vi "Teleop.vi"(10 "Match Info":T1={"Autonomous Elapsed Seconds"=0.0, "TeleOp Elapsed Seconds"=0.0, "Disabled Elapsed Seconds"=0.0, "Visited Autonomous"=FALSE, "Visited TeleOp"=FALSE, "Visited Disabled"=FALSE, "Autonomous Settings"={"Autonomous Style"=enum."Independent", "VI Refnum"=refnum}}, 11 "Call Context":T2) -> ()   [LabVIEW 2013]
doc: "This VI is called for each TeleOp packet received from the DS where the robot is not disabled. It is often used to read from the joysticks and update I/O or to update setpoints for timed control loops. It should complete and return within 20 milliseconds or it may miss DS packets."
uses:
  <vilib>/Rock Robotics/WPI/DriverStation/WPI_DriverStationDerivedRobotMode.ctl
  <vilib>/Rock Robotics/WPI/DriverStation/WPI_DriverStationMatch Info.ctl
  <vilib>/Rock Robotics/WPI/Solenoid/WPI_SolenoidValue.ctl
  Robot Global Data.vi
  <vilib>/Rock Robotics/WPI/Solenoid/Deprecated/WPI_SolenoidGetBool.vi
  <vilib>/Rock Robotics/WPI/Solenoid/WPI_SolenoidSetEnum.vi
  <vilib>/Rock Robotics/WPI/Joystick/WPI_JoystickGetSetRefNum.vi
  <vilib>/Rock Robotics/WPI/RobotDrive/WPI_RobotDriveGetSetRefNum.vi
panel:
  out "Numeric 1":dbl(slide) scale=0.0..100.0
  out "Boolean 2":bool
  out "Boolean 1":bool
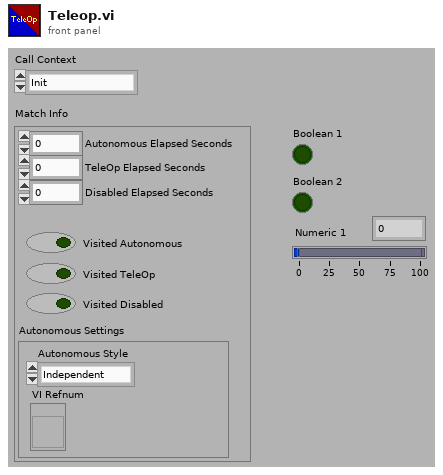
[diagram p1: front panel]
types:
  T1 = typedef "WPI_DriverStationMatch Info.ctl" = cluster{"Autonomous Elapsed Seconds":dbl, "TeleOp Elapsed Seconds":dbl, "Disabled Elapsed Seconds":dbl, "Visited Autonomous":bool, "Visited TeleOp":bool, "Visited Disabled":bool, "Autonomous Settings":cluster{"Autonomous Style":enum16{"Iterative", "Independent"}, "VI Refnum":refnum<vi>}}
  T2 = typedef "WPI_DriverStationDerivedRobotMode.ctl" = enum16{"Init", "Execute", "Stop"}
  T3 = typedef "WPI_JoystickDevRef.ctl" = cluster{"Device":T4}
  T4 = typedef "WPI_JoystickDeviceEnum.ctl" = enum16{"USB 1", "USB 2", "USB 3", "USB 4", "Kinect 1", "Kinect 2"}
  T5 = typedef "WPI_JoystickButtonState.ctl" = cluster{"Button 1":bool, "Button 2":bool, "Button 3":bool, "Button 4":bool, "Button 5":bool, "Button 6":bool, "Button 7":bool, "Button 8":bool, "Button 9":bool, "Button 10":bool, "Button 11":bool, "Button 12":bool}
  T6 = typedef "WPI_SolenoidDevRef.ctl" = cluster{"DevStatus":errorcluster, "Solenoid Module":T7, "Forward Solenoid Channel":T8, "Reverse Solenoid Channel":T8}
  T7 = typedef "FPGA_TypedefSolenoidModule.ctl" = enum16{"Solenoid Module 1", "Solenoid Module 2"}
  T8 = typedef "WPI_SolenoidChannel.ctl" = enum8{"Solenoid 1", "Solenoid 2", "Solenoid 3", "Solenoid 4", "Solenoid 5", "Solenoid 6", "Solenoid 7", "Solenoid 8", "Invalid"}
  T9 = typedef "WPI_SolenoidValue.ctl" = enum16{"Off", "On", "Forward", "Reverse"}
  T10 = typedef "WPI_MotorControlDeviceRef.ctl" = cluster{"DeviceStatus":errorcluster, "Type":enum16{"PWM", "CAN"}, "PWM":cluster{"Digital Module":T11, "PWM Channel":T12, "DeadBand":T13}, "CAN":cluster{"Device Number":u8, "Control Mode":T14, "Semaphore":T15, "Max Vout":dbl}, "Invert":bool, "TransformRef":T16, "InvTransformRef":T16}
  T11 = typedef "FPGA_TypedefDigitalModule.ctl" = enum16{"Digital Module 1", "Digital Module 2"}
  T12 = typedef "FPGA_DIOPWMChannel.ctl" = enum8{"PWM 1", "PWM 2", "PWM 3", "PWM 4", "PWM 5", "PWM 6", "PWM 7", "PWM 8", "PWM 9", "PWM 10", "Invalid"}
  T13 = typedef "WPI_PWMDeadband.ctl" = cluster{"Name":string, "maxPositivePwm":i32, "minPositivePwm":i32, "centerPwm":i32, "maxNegativePwm":i32, "minNegativePwm":i32, "angularRange":u16}
  T14 = typedef "WPI_CANJaguar_ControlMode.ctl" = enum8{"Percent VBus", "Current", "Speed", "Position", "Voltage"}
  T15 = typedef "Semaphore RefNum" = refnum<k1>
  T16 = typedef "WPI_PWMTransform_ConPane.ctl" = refnum<vi>
  T17 = typedef "WPI_RobotDriveDevRef.ctl" = cluster{"DevStatus":errorcluster, "Motors[]":T10[], "Square Inputs":bool, "Max Output":dbl, "Isochronous":bool}
  T18 = cluster{"axis 1 (x)":dbl, "axis 2 (y)":dbl, "axis 3 (throttle)":dbl, "axis 4":dbl, "axis 5":dbl, "axis 6":dbl}
  T19 = typedef "WPI_RelayDevRef.ctl" = cluster{"DevStatus":errorcluster, "Relay Channel":T20, "Digital Module":T11, "Relay Direction":T21}
  T20 = typedef "FPGA_DIORelayChannel.ctl" = enum8{"Relay 1", "Relay 2", "Relay 3", "Relay 4", "Relay 5", "Relay 6", "Relay 7", "Relay 8", "Invalid"}
  T21 = typedef "WPI_RelayDirection.ctl" = enum16{"Both directions", "Forward only", "Reverse only"}
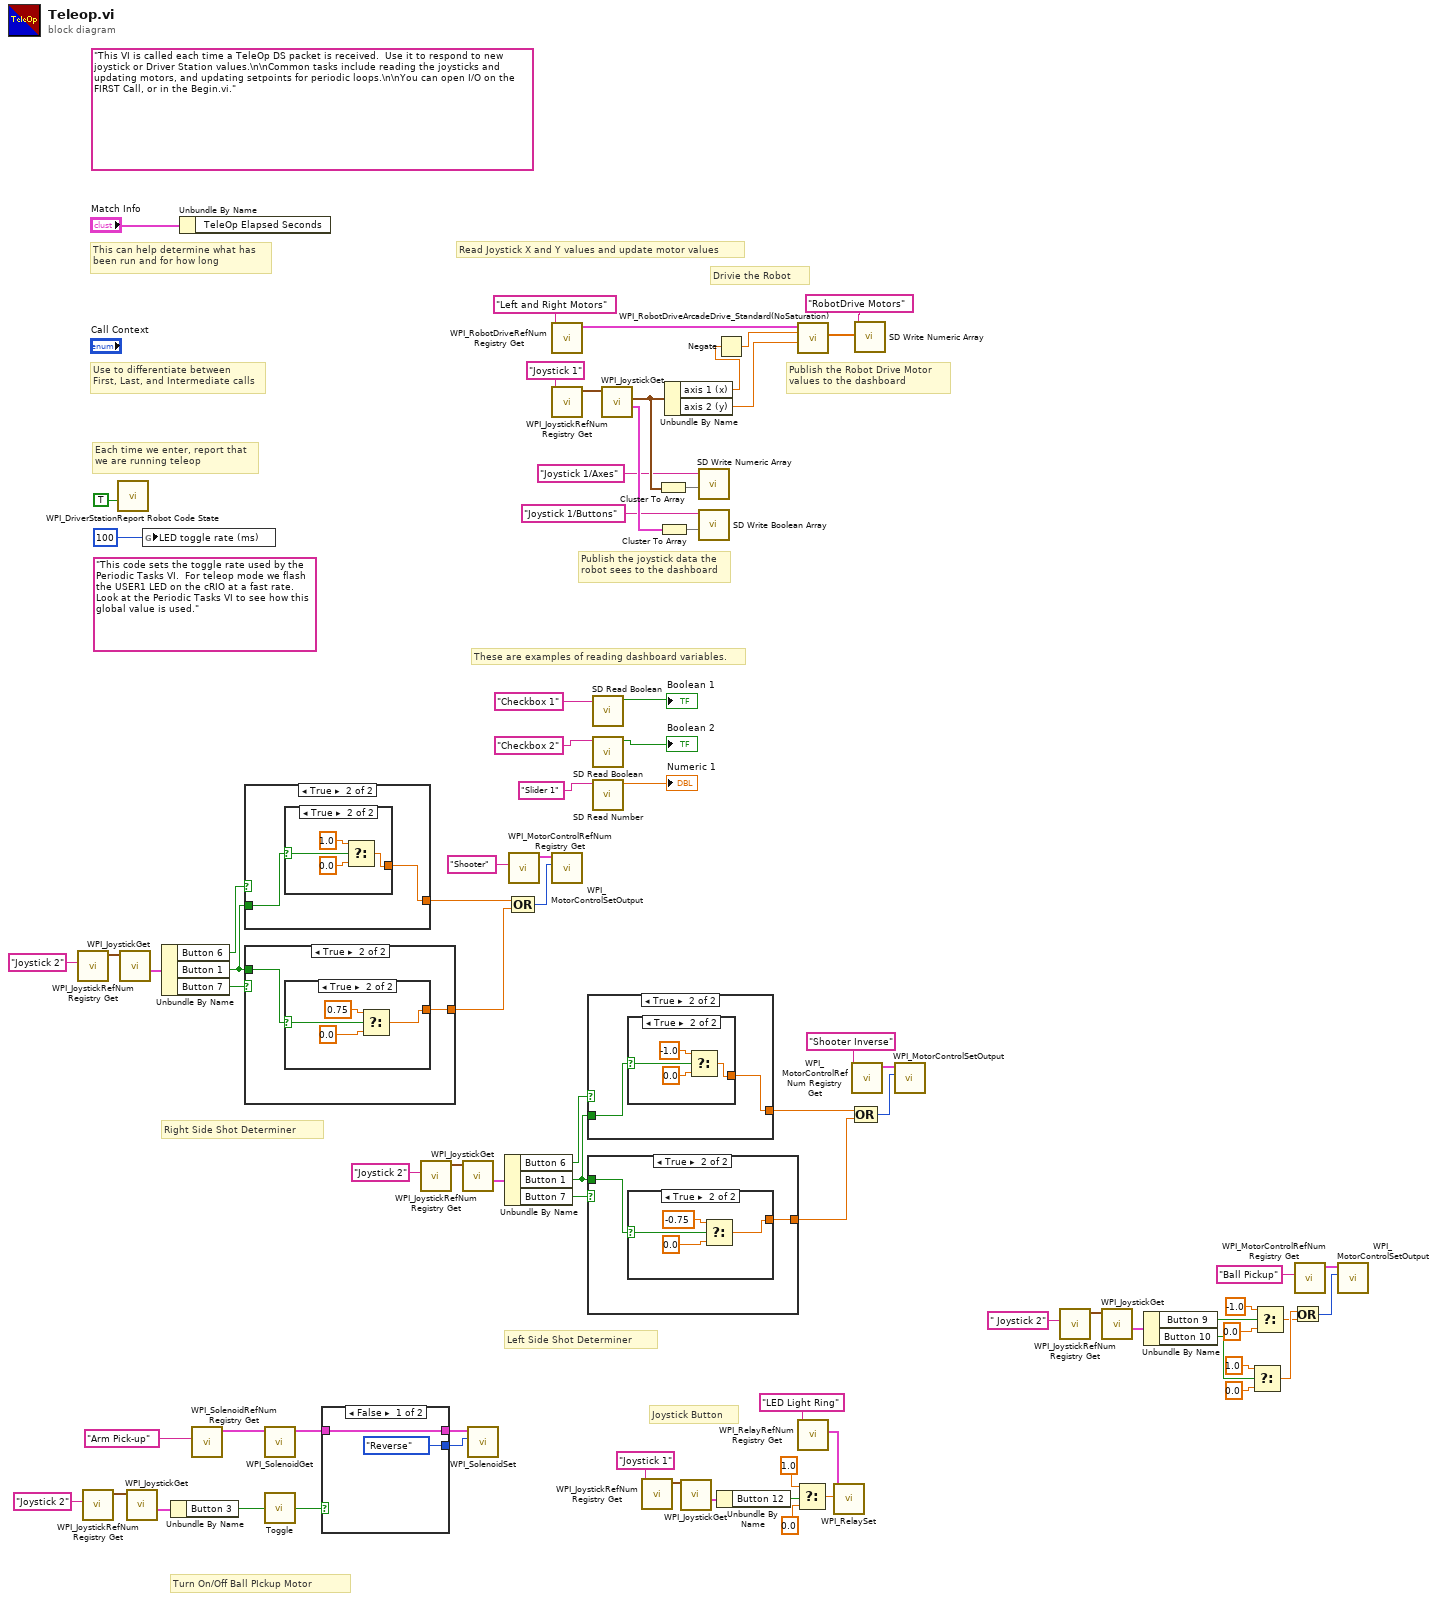
[diagram p0: block diagram]
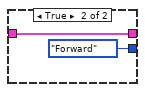
[diagram p2: hidden frame]
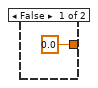
[diagram p3: hidden frame]
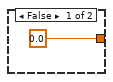
[diagram p4: hidden frame]
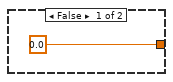
[diagram p5: hidden frame]
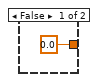
[diagram p6: hidden frame]
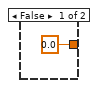
[diagram p7: hidden frame]
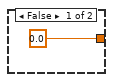
[diagram p8: hidden frame]
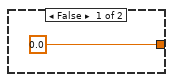
[diagram p9: hidden frame]
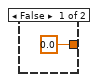
[diagram p10: hidden frame]
diagram:
  (unwired) "This code sets the toggle rate used by the Periodic Tasks VI.  For teleop mode we flash the USER1 LED on the cRIO at a fast rate.  Look at the Periodic Tasks VI to see how this global value is used."
  (unwired) "This VI is called each time a TeleOp DS packet is received.  Use it to respond to new joystick or Driver Station values.\n\nCommon tasks include reading the joysticks and updating motors, and updating setpoints for periodic loops.\n\nYou can open I/O on the FIRST Call, or in the Begin.vi."
  # "Left Side Shot Determiner"
  # "Turn On/Off Ball PIckup Motor"
  # "Right Side Shot Determiner"
  # "Joystick Button"
  # "Drivie the Robot"
  # "These are examples of reading dashboard variables."
  # "Publish the Robot Drive Motor\nvalues to the dashboard"
  # "Publish the joystick data the\nrobot sees to the dashboard"
  # "Each time we enter, report that\nwe are running teleop"
  # "Use to differentiate between\nFirst, Last, and Intermediate calls"
  # "This can help determine what has\nbeen run and for how long"
  # "Read Joystick X and Y values and update motor values"
  n1 = call <vilib>:"WPI_JoystickRefNum Registry Get.vi"("refnum name"="Joystick 2") -> ("JoystickDevRef"=w47:T3)  [unwired: 9 in, 1 out]
  n2 = call <vilib>:"WPI_JoystickRefNum Registry Get.vi"("refnum name"="Joystick 2") -> ("JoystickDevRef"=w41:T3)  [unwired: 9 in, 1 out]
  n3 = call <vilib>:"WPI_DriverStationReport Robot Code State.vi"("TeleOp"=TRUE ("Autonomous")) -> ()  [unwired: 10 in, 1 out]
  n4 = call <vilib>:"WPI_JoystickGet.vi"("JoystickDevRef"=w47) -> ("Buttons"=w46:T5)  [unwired: 4 in, 2 out]
  n5 = call <vilib>:"WPI_JoystickGet.vi"("JoystickDevRef"=w41) -> ("Buttons"=w40:T5)  [unwired: 4 in, 2 out]
  n6 = global write "Robot Global Data.vi" "LED toggle rate (ms)"(u32 100 ("LED ms toggle rate")) -> ()
  n7 = Unbundle By Name(w46) -> ("Button 6"=w36:bool, "Button 1"=w34:bool, "Button 7"=w35:bool)
  n8 = Unbundle By Name(w40) -> ("Button 3"=w37:bool)
  n9 = Unbundle By Name("Match Info") -> ()  [unwired: 1 out]
  n10 = call <vilib>:"WPI_SolenoidRefNum Registry Get.vi"("refnum name"="Arm Pick-up") -> ("SolenoidDevRef"=w5:T6)  [unwired: 9 in, 1 out]
  n11 = case shown="True" w36 {
    tunnel: w34 -> [_ w82]
    tunnel: [0.0 ("f") w81] -> w33
    frame False {
    }
    frame True {
      n12 = case shown="True" w82 {
        selector: w82 -> [_ w85]
        tunnel: [0.0 ("f") w84] -> w81
        frame False {
        }
        frame True {
          n13 = Select(t=1.0, s=w85, f=0.0) -> (s? t:f=w84:dbl)
        }
      }
    }
  }
  n14 = case shown="True" w35 {
    tunnel: w34 -> [_ w90]
    tunnel: [0.0 ("f") w89] -> w32
    frame False {
    }
    frame True {
      n15 = case shown="True" w90 {
        selector: w90 -> [_ w93]
        tunnel: [0.0 ("f") w92] -> w89
        frame False {
        }
        frame True {
          n16 = Select(t=0.75, s=w93, f=0.0) -> (s? t:f=w92:dbl)
        }
      }
    }
  }
  n17 = call-poly <vilib>:"WPI_SolenoidGet.vi"("SolenoidDevRef"=w5) -> ("SolenoidDevRef"=w3:T6)  [unwired: 8 in, 2 out]
  n18 = call "Toggle.vi"("Input"=w37) -> ("Toggled Output"=w4:bool)
  n19 = case shown="False" w4 {
    tunnel: w3 -> [w97 w99]
    tunnel: [w97 w99] -> w2
    tunnel: [WPI_SolenoidValue."Reverse" ("Value") WPI_SolenoidValue."Forward" ("Value")] -> w1
    frame False {
    }
    frame True {
    }
  }
  n20 = call <vilib>:"WPI_JoystickRefNum Registry Get.vi"("refnum name"="Joystick 2") -> ("JoystickDevRef"=w19:T3)  [unwired: 9 in, 1 out]
  n21 = call <vilib>:"WPI_JoystickGet.vi"("JoystickDevRef"=w19) -> ("Buttons"=w20:T5)  [unwired: 4 in, 2 out]
  n22 = call-poly <vilib>:"WPI_SolenoidSet.vi"("Value"=w1, "SolenoidDevRef"=w2) -> ()  [unwired: 8 in, 2 out]
  n23 = Unbundle By Name(w20) -> ("Button 6"=w21:bool, "Button 1"=w23:bool, "Button 7"=w22:bool)
  n24 = call <vilib>:"WPI_MotorControlRefNum Registry Get.vi"("refnum name"="Shooter") -> ("MotorControlDevRef"=w29:T10)  [unwired: 9 in, 1 out]
  n25 = Compound Arithmetic op=OR(w33, w32) -> (w31:i32)
  n26 = call <vilib>:"WPI_RobotDriveRefNum Registry Get.vi"("refnum name"="Left and Right Motors") -> ("RobotDriveDevRef"=w77:T17)  [unwired: 1 in, 9 out]
  n27 = call <vilib>:"WPI_JoystickRefNum Registry Get.vi"("refnum name"="Joystick 1") -> ("JoystickDevRef"=w74:T3)  [unwired: 1 in, 9 out]
  n28 = call <vilib>:"WPI_MotorControlSetOutput.vi"("Output"=w31, "MotorControlDevRef"=w29) -> ()  [unwired: 7 in, 3 out]
  n29 = case shown="True" w21 {
    tunnel: w23 -> [_ w102]
    tunnel: [0.0 ("f") w101] -> w24
    frame False {
    }
    frame True {
      n30 = case shown="True" w102 {
        selector: w102 -> [_ w105]
        tunnel: [0.0 ("f") w104] -> w101
        frame False {
        }
        frame True {
          n31 = Select(t=-1.0, s=w105, f=0.0) -> (s? t:f=w104:dbl)
        }
      }
    }
  }
  n32 = case shown="True" w22 {
    tunnel: w23 -> [_ w110]
    tunnel: [0.0 ("f") w109] -> w25
    frame False {
    }
    frame True {
      n33 = case shown="True" w110 {
        selector: w110 -> [_ w113]
        tunnel: [0.0 ("f") w112] -> w109
        frame False {
        }
        frame True {
          n34 = Select(t=-0.75, s=w113, f=0.0) -> (s? t:f=w112:dbl)
        }
      }
    }
  }
  n35 = call <vilib>:"SD Read Boolean.vi"("Name"="Checkbox 1" ("refnum name")) -> ("Boolean"=→"Boolean 1":bool)  [unwired: 8 in, 2 out]
  n36 = call <vilib>:"SD Read Boolean.vi"("Name"="Checkbox 2" ("refnum name")) -> ("Boolean"=→"Boolean 2":bool)  [unwired: 8 in, 2 out]
  n37 = call <vilib>:"SD Read Number.vi"("Name"="Slider 1" ("refnum name")) -> ("Numeric"=→"Numeric 1":dbl)  [unwired: 8 in, 2 out]
  n38 = call <vilib>:"WPI_JoystickGet.vi"("JoystickDevRef"=w74) -> ("Buttons"=w71:T5, "Axes"=w68:T18)  [unwired: 1 in, 4 out]
  n39 = call <vilib>:"WPI_JoystickRefNum Registry Get.vi"("refnum name"="Joystick 1") -> ("JoystickDevRef"=w53:T3)  [unwired: 9 in, 1 out]
  n40 = Cluster To Array(cluster=w68) -> (array=w67:dbl[])
  n41 = Cluster To Array(cluster=w71) -> (array=w70:bool[])
  n42 = Unbundle By Name(w68) -> ("axis 1 (x)"=w39:dbl, "axis 2 (y)"=w76:dbl)
  n43 = call <vilib>:"WPI_JoystickGet.vi"("JoystickDevRef"=w53) -> ("Buttons"=w52:T5)  [unwired: 4 in, 2 out]
  n44 = call <vilib>:"SD Write Numeric Array.vi"("Numeric Array"=w67, "Name"="Joystick 1/Axes") -> ()  [unwired: 8 in, 2 out]
  n45 = call <vilib>:"SD Write Boolean Array.vi"("Boolean Array"=w70, "Name"="Joystick 1/Buttons") -> ()  [unwired: 8 in, 2 out]
  n46 = Negate(x=w39) -> (-x=w38:dbl)
  n47 = Unbundle By Name(w52) -> ("Button 12"=w51:bool)
  n48 = Select(t=1.0, s=w51, f=0.0) -> (s? t:f=w50:dbl)
  n49 = call <vilib>:"WPI_RobotDriveArcadeDrive_Standard(NoSaturation).vi"("Y axis value"=w76, "X axis value"=w38, "RobotDriveDevRef"=w77) -> ("Motor Values"=w64:dbl[])  [unwired: 1 in, 7 out]
  n50 = call <vilib>:"WPI_RelayRefNum Registry Get.vi"("refnum name"="LED Light Ring") -> ("RelayDevRef"=w57:T19)  [unwired: 9 in, 1 out]
  n51 = call <vilib>:"WPI_RelaySet.vi"("RelayValue"=w50, "RelayDevRef"=w57) -> ()  [unwired: 8 in, 2 out]
  n52 = call <vilib>:"WPI_MotorControlRefNum Registry Get.vi"("refnum name"="Shooter Inverse") -> ("MotorControlDevRef"=w28:T10)  [unwired: 9 in, 1 out]
  n53 = call <vilib>:"SD Write Numeric Array.vi"("Numeric Array"=w64, "Name"="RobotDrive Motors") -> ()  [unwired: 8 in, 2 out]
  n54 = Compound Arithmetic op=OR(w24, w25) -> (w26:i32)
  n55 = call <vilib>:"WPI_MotorControlSetOutput.vi"("Output"=w26, "MotorControlDevRef"=w28) -> ()  [unwired: 7 in, 3 out]
  n56 = call <vilib>:"WPI_JoystickRefNum Registry Get.vi"("refnum name"=" Joystick 2") -> ("JoystickDevRef"=w11:T3)  [unwired: 9 in, 1 out]
  n57 = call <vilib>:"WPI_JoystickGet.vi"("JoystickDevRef"=w11) -> ("Buttons"=w12:T5)  [unwired: 4 in, 2 out]
  n58 = Unbundle By Name(w12) -> ("Button 9"=w13:bool, "Button 10"=w9:bool)
  n59 = Select(t=1.0, s=w9, f=0.0) -> (s? t:f=w8:dbl)
  n60 = Select(t=-1.0, s=w13, f=0.0) -> (s? t:f=w7:dbl)
  n61 = Or(x=w8, y=w7) -> (x .or. y?=w6:i32)
  n62 = call <vilib>:"WPI_MotorControlRefNum Registry Get.vi"("refnum name"="Ball Pickup") -> ("MotorControlDevRef"=w44:T10)  [unwired: 9 in, 1 out]
  n63 = call <vilib>:"WPI_MotorControlSetOutput.vi"("Output"=w6, "MotorControlDevRef"=w44) -> ()  [unwired: 7 in, 3 out]
